vi "Create Table.vi"(8 "error in (no error)":errorcluster) -> (0 "error out":errorcluster)   [LabVIEW 2020, in "Settings.lvlib"]
uses:
  Settings.lvlib
  <vilib>/drjdpowell/SQLite Library/SQL Connection/Open (path).vi
  <vilib>/drjdpowell/SQLite Library/SQL Connection/Open (string).vi
  <vilib>/AdvancedString/Path To Command Line String.vi
  <vilib>/drjdpowell/SQLite Library/SQL Connection/Execute SQL (No results).vi
  <vilib>/drjdpowell/SQLite Library/SQL Connection/Connection.lvclass
  <vilib>/drjdpowell/SQLite Library/SQLite.lvlib
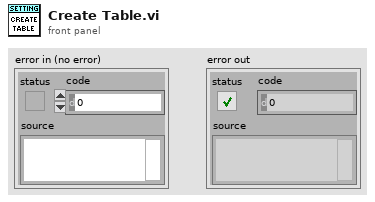
[diagram p1: front panel]
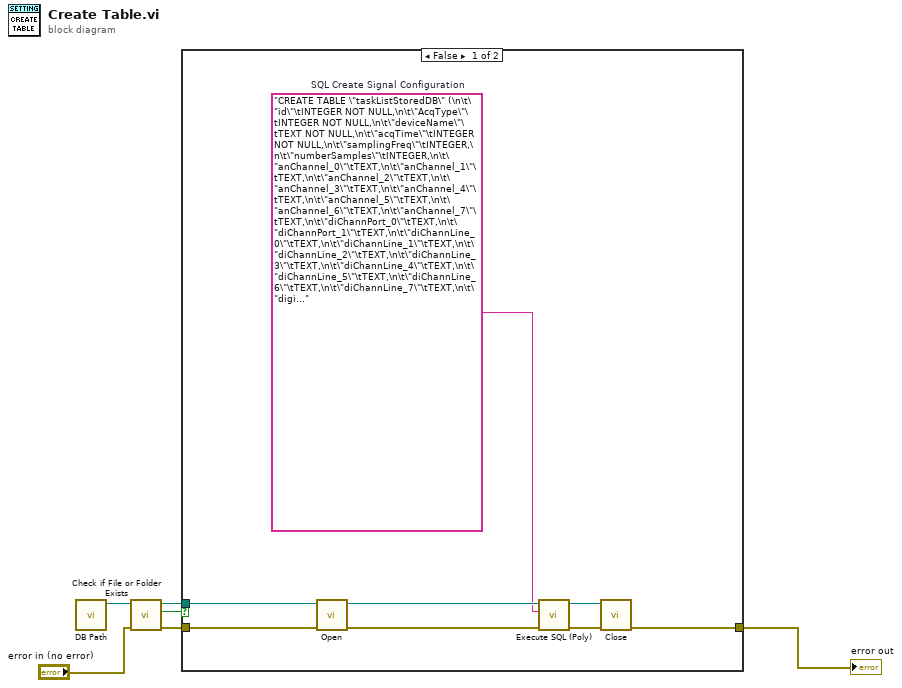
[diagram p0: block diagram]
diagram:
  n1 = call "DB Path.vi"() -> ("DB Path"=w1:path)  [unwired: 11 in]
  n2 = call <vilib>:"Check if File or Folder Exists.vi"("error in (no error)"="error in (no error)", "path"=w1) -> ("error out"=w4:errorcluster, "file or folder exists?"=w2:bool, "dup path"=w6:path)  [unwired: 7 in]
  n3 = case shown="False" w2 {
    tunnel: w6 -> [w10 _]
    tunnel: w4 -> [w9 w15]
    tunnel: [w8 w15] -> w3
    frame False {
      w7 = "CREATE TABLE \"taskListStoredDB\" (\n\t\"id\"\tINTEGER NOT NULL,\n\t\"AcqType\"\tINTEGER NOT NULL,\n\t\"deviceName\"\tTEXT NOT NULL,\n\t\"acqTime\"\tINTEGER NOT NULL,\n\t\"samplingFreq\"\tINTEGER,\n\t\"numberSamples\"\tINTEGER,\n\t\"anChannel_0\"\tTEXT,\n\t\"anChannel_1\"\tTEXT,\n\t\"anChannel_2\"\tTEXT,\n\t\"anChannel_3\"\tTEXT,\n\t\"anChannel_4\"\tTEXT,\n\t\"anChannel_5\"\tTEXT,\n\t\"anChannel_6\"\tTEXT,\n\t\"anChannel_7\"\tTEXT,\n\t\"diChannPort_0\"\tTEXT,\n\t\"diChannPort_1\"\tTEXT,\n\t\"diChannLine_0\"\tTEXT,\n\t\"diChannLine_1\"\tTEXT,\n\t\"diChannLine_2\"\tTEXT,\n\t\"diChannLine_3\"\tTEXT,\n\t\"diChannLine_4\"\tTEXT,\n\t\"diChannLine_5\"\tTEXT,\n\t\"diChannLine_6\"\tTEXT,\n\t\"diChannLine_7\"\tTEXT,\n\t\"digiFreq\"\tINTEGER,\n\t\"portOrLine\"\tINTEGER,\n\tPRIMARY KEY(\"id\" AUTOINCREMENT)\n);"  # SQL Create Signal Configuration
      n4 = call-poly <vilib>:"Open.vi"("error in (no error)"=w9, "db file"=w10) -> ("error out"=w13:errorcluster, "SQLite Connection"=w14:refnum<class "Connection.lvclass">)  [unwired: 8 in]
      n5 = call-poly <vilib>:"Execute SQL (Poly).vi"("error in (no error)"=w13, "SQL"=w7, "SQLite Connection in"=w14) -> ("error out"=w11:errorcluster, "SQLite Connection"=w12:refnum<class "Connection.lvclass">)  [unwired: 7 in]
      n6 = call-dynamic "Close.vi"("error in (no error)"=w11, "SQLite Connection in"=w12) -> ("error out"=w8:errorcluster)  [unwired: 9 in]
    }
    frame True {
    }
  }
  "error out" <- w3
